vi "Initialize NodeBrowserWF.vi"(7 "Generate?":bool, 8 "error in (no error)":errorcluster, 9 "Output Channels":T2[](array[typedef]) {"Data Type" items=["Signed", "Unsigned", "IEEE Float"]}, 10 "Node Pointer":T1, 11 "NodeBrowserRefs":refnum<k24>[](array[refnum])) -> (0 "error out":errorcluster, 2 "Node Pointer":T1, 3 "NodeBrowserRefs":refnum<k24>[](array[refnum]))   [LabVIEW 2016, in "LIN Frame Protection Addon System Explorer.lvlib"]
uses:
  LIN Frame Protection Addon System Explorer.lvlib
  Shared/Types/InputChannelConfiguration.ctl
  <vilib>/NI Veristand/Custom Device API/Custom Device Pointer.ctl
  NationalInstruments.VeriStand.SystemStorage
  NationalInstruments.VeriStand.SystemStorageUI
  NationalInstruments.VeriStand
  Shared/LIN Frame Protection Addon Shared.lvlib
  <vilib>/NI Veristand/Custom Device API/Custom Device API.lvlib
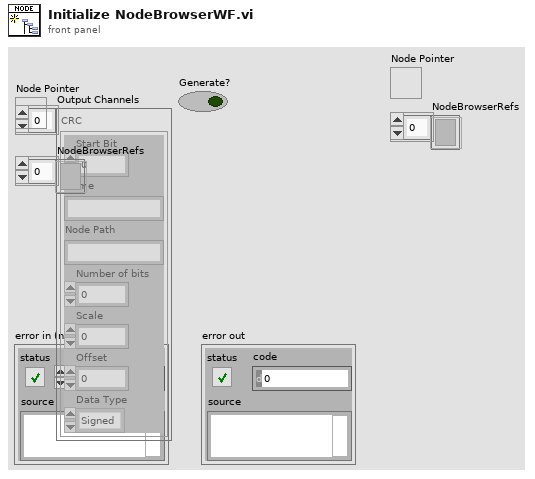
[diagram p1: front panel]
types:
  T1 = typedef "Custom Device API.lvlib/Custom Device Pointer.ctl" = refnum<k24>
  T2 = typedef "LIN Frame Protection Addon Shared.lvlib/InputChannelConfiguration.ctl" = cluster{"Start Bit":i32, "Name":string, "Node Path":string, "Number of bits":i32, "Scale":dbl, "Offset":dbl, "Data Type":u32}
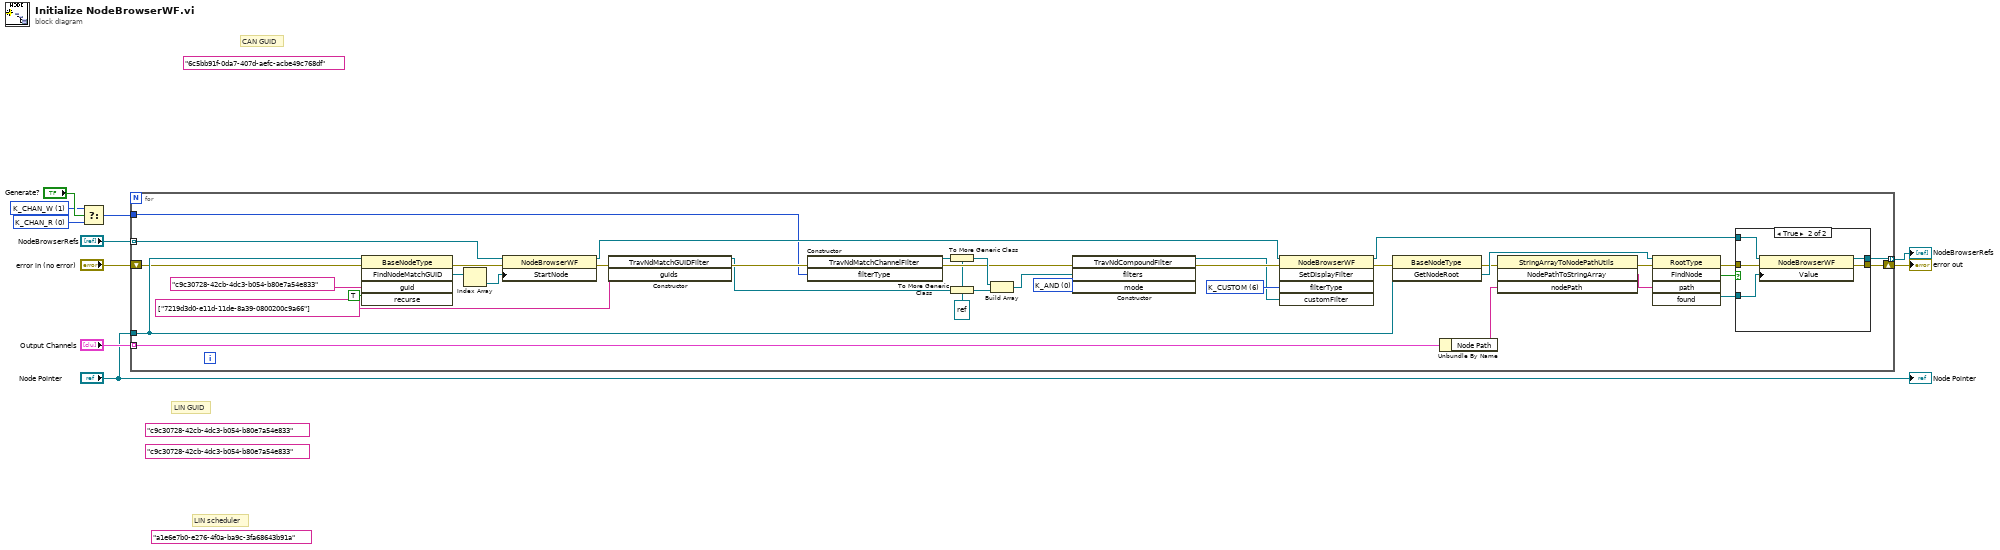
[diagram p0: block diagram]
diagram:
  (unwired) "c9c30728-42cb-4dc3-b054-b80e7a54e833" ("guid")
  (unwired) "a1e6e7b0-e276-4f0a-ba9c-3fa68643b91a" ("guid")
  (unwired) "6c5bb91f-0da7-407d-aefc-acbe49c768df" ("guid")
  (unwired) "c9c30728-42cb-4dc3-b054-b80e7a54e833" ("guid")
  w2 = u8 0 items=["K_CHAN_R", "K_CHAN_W", "K_CHAN_VOLT", "K_CHAN_FAULT"] ("filterType")
  w3 = u8 1 items=["K_CHAN_R", "K_CHAN_W", "K_CHAN_VOLT", "K_CHAN_FAULT"] ("filterType")
  # "LIN scheduler"
  # "LIN GUID"
  # "CAN GUID"
  n1 = Select(t=w3, s="Generate?", f=w2) -> (s? t:f=w4:u8)
  n2 = for {
    tunnel: "NodeBrowserRefs" -> [w47] mode=indexing
    tunnel: [w38] -> w6 mode=indexing
    tunnel: "Node Pointer" -> [w30]
    shift-right: [w37] -> w10
    shift-left: "error in (no error)" -> [w27]
    tunnel: "Output Channels" -> [w36] mode=indexing
    tunnel: w4 -> [w11]
    w15 = refnum<k24> refnum
    w22 = 0 items=["K_AND", "K_OR"] ("mode")
    w34 = u8 6 items=["K_CHAN_R", "K_CHAN_W", "K_CHAN_RW", "K_CHAN_VOLT", "K_CHAN_FAULT", "K_ALL", "K_CUSTOM", "K_CHAN_R_VIS", "K_CHAN_W_VIS", "K_CHAN_RW_VIS", "K_CHAN_VOLT_VIS", "K_CHAN_FAULT_VIS", "K_WAVE", "K_WAVE_VIS", "K_WAVE_DBL", "K_WAVE_CDB", "K_WAVE_DBL_VIS", "K_WAVE_CDB_VIS"] ("filterType")
    n3 = invoke class="BaseNodeType" method="FindNodeMatchGUID"(reference=w30, error in=w27, "guid"="c9c30728-42cb-4dc3-b054-b80e7a54e833", "recurse"=TRUE) -> (error out=w26:errorcluster, "FindNodeMatchGUID"=w29:refnum<k24>[])  [unwired: 1 in, 3 out]
    n4 = Index Array(array=w29) -> (element=w28:refnum<k24>)  [unwired: 1 in]
    n5 = property class="NodeBrowserWF"(reference=w47, error in=w26, "StartNode"=w28) -> (reference out=w12:refnum<k24>, error out=w32:errorcluster)
    n6 = constructor class="TravNdMatchGUIDFilter"(error in=w32, "guids"=string[] ["7219d3d0-e11d-11de-8a39-0800200c9a66"]) -> (reference out=w16:refnum<k24>, error out=w23:errorcluster)  [unwired: 2 in, 2 out]
    n7 = constructor class="TravNdMatchChannelFilter"(error in=w23, "filterType"=w11) -> (reference out=w14:refnum<k24>, error out=w17:errorcluster)  [unwired: 2 in, 2 out]
    n8 = To More Generic Class(target class=w15, reference=w14) -> (generic class reference=w20:refnum<k24>)
    n9 = To More Generic Class(target class=w15, reference=w16) -> (generic class reference=w21:refnum<k24>)
    n10 = Build Array(w20, w21) -> (w19:refnum<k24>[])
    n11 = constructor class="TravNdCompoundFilter"(error in=w17, "filters"=w19, "mode"=w22) -> (reference out=w13:refnum<k24>, error out=w18:errorcluster)  [unwired: 2 in, 3 out]
    n12 = invoke class="NodeBrowserWF" method="SetDisplayFilter"(reference=w12, error in=w18, "filterType"=w34, "customFilter"=w13) -> (reference out=w46:refnum<k24>, error out=w40:errorcluster)  [unwired: 1 in, 3 out]
    n13 = invoke class="BaseNodeType" method="GetNodeRoot"(reference=w30, error in=w40) -> (error out=w44:errorcluster, "GetNodeRoot"=w45:refnum<k24>)  [unwired: 1 in, 1 out]
    n14 = Unbundle By Name(w36) -> ("Node Path"=w35:string)
    n15 = invoke class="StringArrayToNodePathUtils" method="NodePathToStringArray"(error in=w44, "nodePath"=w35) -> (error out=w42:errorcluster, "NodePathToStringArray"=w43:string[])  [unwired: 2 in, 2 out]
    n16 = invoke class="RootType" method="FindNode"(reference=w45, error in=w42, "path"=w43) -> (error out=w39:errorcluster, "FindNode"=w33:bool, "found"=w41:refnum<k24>)  [unwired: 2 in, 2 out]
    n17 = case shown="True" w33 {
      tunnel: w46 -> [w48 w54]
      tunnel: w41 -> [_ w53]
      tunnel: w39 -> [w49 w52]
      tunnel: [w48 w51] -> w38
      tunnel: [w49 w50] -> w37
      frame False {
      }
      frame True {
        n18 = property class="NodeBrowserWF"(reference=w54, error in=w52, "Value"=w53) -> (reference out=w51:refnum<k24>, error out=w50:errorcluster)
      }
    }
  }
  "error out" <- w10
  "NodeBrowserRefs" <- w6
  "Node Pointer" <- "Node Pointer"
